vi "Read Queued Processed Outgoing Messages.vi"(6 "timeout in ms (-1)":i32=100, 8 "error in":errorcluster, 11 "j1939 queues":T1) -> (0 "error out":errorcluster, 2 "timed out?":bool, 3 "Frames":T2[](array[typedef]) {"Identifier" format="%08x"})   [LabVIEW 2013, in "J1939.lvlib"]
uses:
  J1939.lvlib
  API Types/CAN Outgoing Message Cluster.ctl
  API Types/Setup Information Cluster.ctl
  API Types/Convert DTCs Cluster.ctl
  <vilib>/xnet/xnet.llb/XNET Frame CAN.ctl
  <vilib>/xnet/xnet.llb/XNET Frame Type CAN.ctl
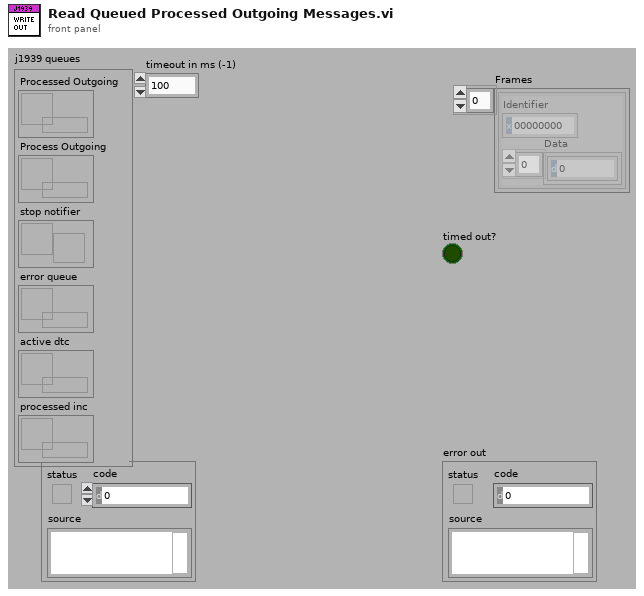
[diagram p1: front panel]
types:
  T1 = typedef "J1939.lvlib/Setup Information Cluster.ctl" = cluster{"Processed Outgoing":refnum<queue>, "Process Outgoing":refnum<queue>, "stop notifier":refnum<notifier>, "error queue":refnum<queue>, "active dtc":refnum<queue>, "processed inc":refnum<queue>}
  T2 = typedef "J1939.lvlib/CAN Outgoing Message Cluster.ctl" = cluster{"Identifier":u32, "Data":u8[]}
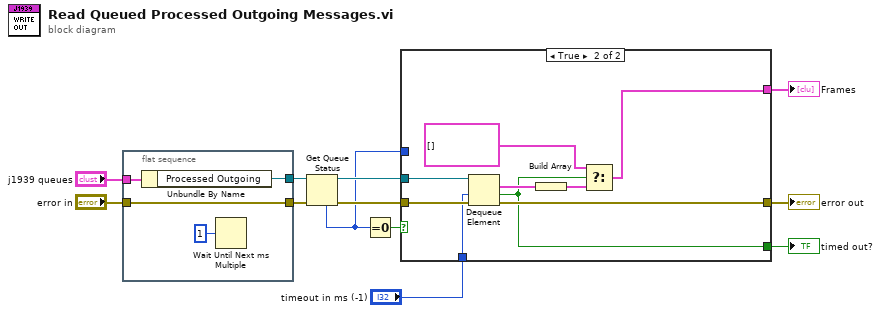
[diagram p0: block diagram]
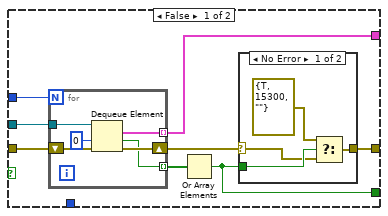
[diagram p2: hidden frame]
diagram:
  n1 = flat-sequence {
    tunnel: [w16] -> w8
    tunnel: "j1939 queues" -> [w15]
    tunnel: [w13] -> w4
    tunnel: "error in" -> [w13]
    frame #0 {
      n2 = Unbundle By Name(w15) -> ("Processed Outgoing"=w16:refnum<queue>)
      n3 = Wait Until Next ms Multiple(millisecond multiple=u32 1) -> ()  [unwired: 1 out]
    }
  }
  n4 = Get Queue Status(queue=w8, error in (no error)=w4) -> (queue out=w12:refnum<queue>, error out=w11:errorcluster, # elements in queue=w9:i32)  [unwired: 6 out]
  n5 = Equal To 0?(x=w9) -> (x = 0?=w10:bool)
  n6 = case shown="True" w10 {
    tunnel: [w18 w42] -> w6
    tunnel: w12 -> [w24 w44]
    tunnel: w11 -> [w22 w43]
    tunnel: [w23 w39] -> w7
    tunnel: w9 -> [w21 _]
    tunnel: [w19 w37] -> w5
    tunnel: "timeout in ms (-1)" -> [_ w36]
    frame False {
      n7 = for {
        N: w21 -> [_]
        tunnel: w24 -> [w34]
        tunnel: [w33] -> w23 mode=indexing
        shift-right: [w35] -> w17
        shift-left: w22 -> [w32]
        tunnel: [w31] -> w20 mode=indexing
        n8 = Dequeue Element(queue=w34, timeout in ms (-1)=0, error in (no error)=w32) -> (element=w33:T2, timed out?=w31:bool, error out=w35:errorcluster)  [unwired: 1 out]
      }
      n9 = Or Array Elements(Boolean array=w20) -> (logical OR=w19:bool)
      n10 = case shown="No Error" w17 {
        selector: w17 -> [w25 w29]
        tunnel: w19 -> [w28 _]
        tunnel: [w27 w29] -> w18
        frame No Error {
          n11 = Select(t=errorcluster {"status"=TRUE, "code"=15300, "source"=""}, s=w28, f=w25) -> (s? t:f=w27:errorcluster)
        }
        frame Error {
        }
      }
    }
    frame True {
      n12 = Dequeue Element(queue=w44, timeout in ms (-1)=w36, error in (no error)=w43) -> (element=w41:T2, timed out?=w37:bool, error out=w42:errorcluster)  [unwired: 1 out]
      n13 = Build Array(w41) -> (w40:T2[])
      n14 = Select(t=T2[] [], s=w37, f=w40) -> (s? t:f=w39:T2[])
    }
  }
  "Frames" <- w7
  "error out" <- w6
  "timed out?" <- w5
